vi "TestDAQOrcaFlash.vi"   [LabVIEW 2012]
uses:
  DAQOrcaFlash/DAQOrcaFlash.lvclass
  <vilib>/Distrio/Murmex/Murmex/Murmex.lvclass
panel:
  # "Test DAQ"
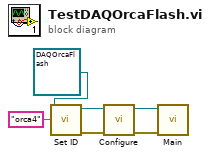
[diagram p0: block diagram]
diagram:
  n1 = call <vilib>:"Set ID.vi"("id"="orca4", "Murmex in"=refnum<class "DAQOrcaFlash.lvclass"> refnum ("DAQOrcaFlash.lvclass")) -> ("error out"=w2:errorcluster, "Murmex out"=w5:refnum<class "DAQOrcaFlash.lvclass">)  [unwired: 8 in]
  n2 = call-dynamic "Configure.vi"("error in (no error)"=w2, "DAQMH121119OrcaFlash in"=w5) -> ("error out"=w1:errorcluster, "DAQMH121119OrcaFlash out"=w3:refnum<class "DAQOrcaFlash.lvclass">)  [unwired: 7 in, 1 out]
  n3 = call-dynamic "Main.vi"("error in (no error)"=w1, "DAQMH121119OrcaFlashBase in"=w3) -> ()  [unwired: 8 in, 2 out]
